vi "setSweepTime.vi"(8 "error in (no error)":errorcluster, 10 "Sweep Time (s)":dbl, 11 "Instrument.LockinAPI in":refnum<class "Instrument.LockinAPI.lvclass">) -> (0 "error out":errorcluster, 3 "Instrument.LockinAPI out":refnum<class "Instrument.LockinAPI.lvclass">)   [LabVIEW 2019, in "Instrument.LockinAPI.lvclass"]
doc: "API to set Sweep Time"
uses:
  Instrument.LockinAPI.lvclass
  C:/Users/patrick/Documents/GitHub/Instrument-Framework/lvsrc/Instrument/Instrument.lvclass
  Typedefs/API/LockinAPI.Commands--Enum.ctl
  de6fb303-8df8-49ef-b17e-c3f9f1bf9765.vi
  de6fb303-8df8-49ef-b17e-c3f9f1bf9765.vi/95c2deb2-50ee-4984-8800-0334412be20b.vi
  de6fb303-8df8-49ef-b17e-c3f9f1bf9765.vi/95c2deb2-50ee-4984-8800-0334412be20b.vi/6e451b3b-cbe6-4375-87f8-2e681efdab37.vi
  de6fb303-8df8-49ef-b17e-c3f9f1bf9765.vi/95c2deb2-50ee-4984-8800-0334412be20b.vi/b9c0e159-9ef2-4bae-9ebc-0760e0319bea.vi
  de6fb303-8df8-49ef-b17e-c3f9f1bf9765.vi/95c2deb2-50ee-4984-8800-0334412be20b.vi/9776c926-d2f5-4942-a4e3-21116c5d8f60.vi
  <vilib>/JDP Science/JSONtext/Make JSON Array.vi
  de6fb303-8df8-49ef-b17e-c3f9f1bf9765.vi/95c2deb2-50ee-4984-8800-0334412be20b.vi/b9c0e159-9ef2-4bae-9ebc-0760e0319bea.vi/7f334bb6-daaa-4c89-80ee-cf0ecf440f19.vi
  de6fb303-8df8-49ef-b17e-c3f9f1bf9765.vi/95c2deb2-50ee-4984-8800-0334412be20b.vi/9776c926-d2f5-4942-a4e3-21116c5d8f60.vi/f76175da-9965-4863-9bcc-ee9f29f0bb01.vi
  de6fb303-8df8-49ef-b17e-c3f9f1bf9765.vi/95c2deb2-50ee-4984-8800-0334412be20b.vi/9776c926-d2f5-4942-a4e3-21116c5d8f60.vi/dd00b1fc-4702-4092-afca-377c266024ee.vi
  Instrument/API/Enum to String.vi
  Instrument/Private/Get RC Connection Status.vi
  <vilib>/JDP Science/JSONtext/Variant to JSON Text.vi
  <vilib>/JDP Science/JSONtext/support/Format JSON Array Text.vi
  Instrument/API/Send and Receive.vi
  <vilib>/JDP Science/JSONtext/JSON text to Variant.vi
  <vilib>/Utility/Data Type/Get Type Information.vi
  <vilib>/JDP Science/JSONtext/LVClass Serializer/JSONtext LVClass Serializer.lvclass
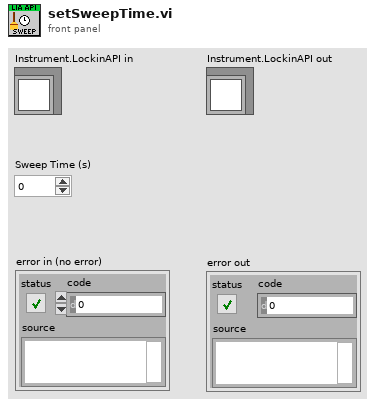
[diagram p1: front panel]
types:
  T1 = typedef "Instrument.LockinAPI.lvclass/LockinAPI.Commands--Enum.ctl" = enum16{"setAI", "setAO", "setAO_Amplitude", "setAO_DC", "setAO_Frequency", "setAO_Phase", "setAO_Function", "setAO_I+", "setREF", "setREF_Frequency", "setREF_Phase", "setREF_TC", "setREF_Roll-Off", "setDAQ", "setSampling", "setOffset", "setState", "getState", "getAO", "getAI", "getResults", "getSampling", "getAOconfig", "getREFconfig", "setInputGain", "setOutputGain", "getInputGain", "getOutputGain", "setSamplingMode", "getSamplingMode", "setSweep", "setSweepTime", "setSweepTable", "getStatus", "getSweepResults", "getSweepWaveforms", "startSweep", "stopSweep", "setAUX", "getAUX"}
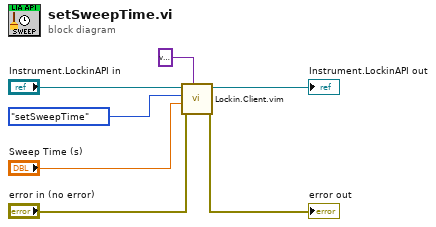
[diagram p0: block diagram]
diagram:
  n1 = call "Lockin.Client.vim"("Data Out type"=variant, "error in (no error)"="error in (no error)", "Data"="Sweep Time (s)", "Command"=LockinAPI.Commands--Enum."setSweepTime", "Instrument.LockinAPI in"="Instrument.LockinAPI in") -> ("error out"=→"error out":errorcluster, "Instrument.LockinAPI out"=→"Instrument.LockinAPI out":refnum<class "Instrument.LockinAPI.lvclass">)  [unwired: 4 in, 1 out]
